vi "OPCUA Disconnect.vi"(8 "error in (no error)":errorcluster, 11 "reference":refnum<k24>) -> (0 "error out":errorcluster, 3 "reference out":refnum<k24>)   [LabVIEW 2019]
uses:
  F:/src/HUTCDLSVN/Machine/CDL0100/TagEngine/LVOPCUA.NET/LVOPC.NETInterface/bin/Release/LVOPC.NETInterface.dll
  LVOPCUA.NET/LVOPC.NETInterface/bin/Release/LVOPC.NETInterface.dll
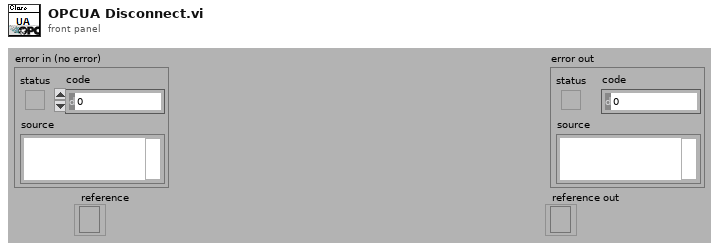
[diagram p1: front panel]
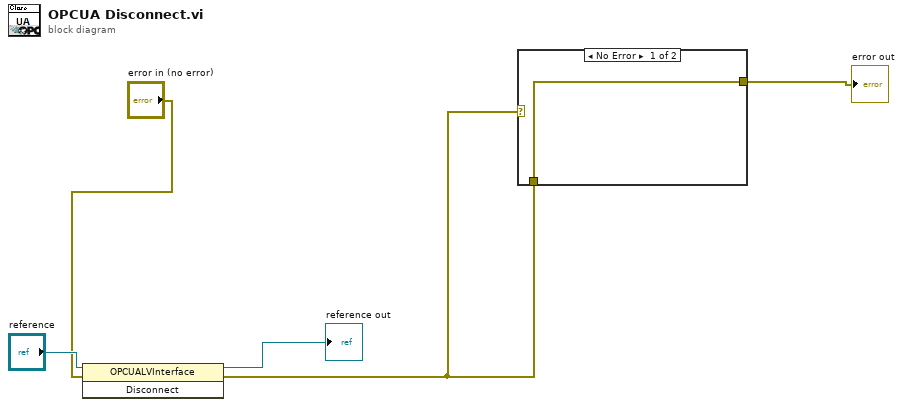
[diagram p0: block diagram]
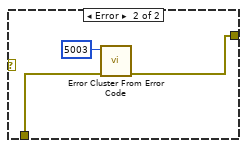
[diagram p2: hidden frame]
diagram:
  n1 = invoke class="OPCUALVInterface" method="Disconnect"(reference="reference", error in="error in (no error)") -> (reference out=→"reference out":refnum<k24>, error out=w1:errorcluster)  [unwired: 1 in, 1 out]
  n2 = case shown="No Error" w1 {
    tunnel: [w6 w8] -> w5
    tunnel: w1 -> [w6 w7]
    frame No Error {
    }
    frame Error {
      n3 = call <vilib>:"Error Cluster From Error Code.vi"("error in (no error)"=w7, "error code (0)"=5003) -> ("error out"=w8:errorcluster)  [unwired: 7 in]
    }
  }
  "error out" <- w5
